vi "FIFORequests.vi"(1 "Log":T1, 3 "Requests in":T1[](array[typedef])) -> (0 "Requests out":T1[](array[typedef]))   [LabVIEW 2010]
uses:
  _ROSDefinition.vi
  Console/Servers/ServerSubs/ROSLog.ctl
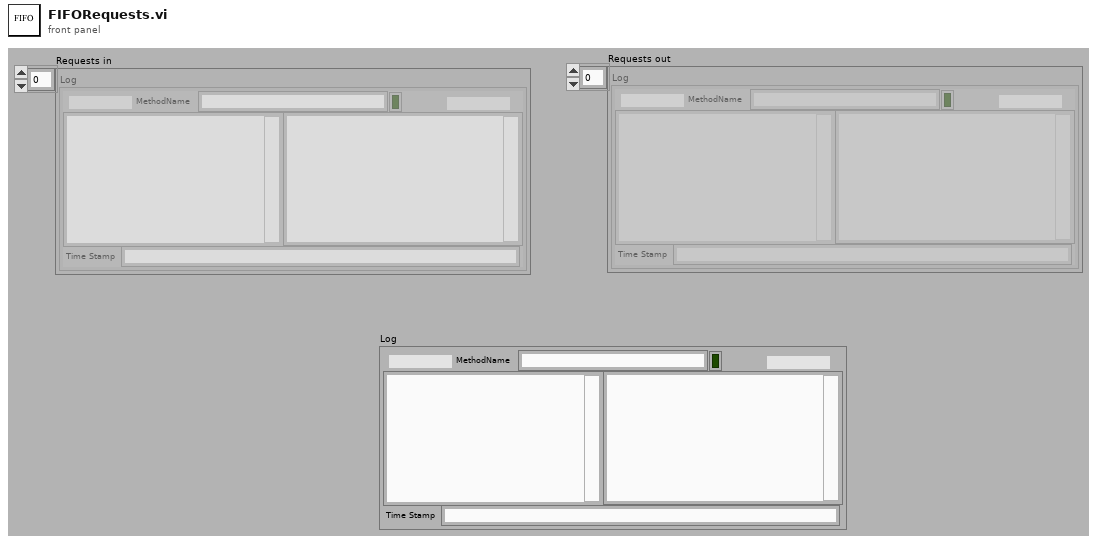
[diagram p1: front panel]
types:
  T1 = typedef "ROSLog.ctl" = cluster{"Sent":string, "Reply":string, "MethodName":string, "success":bool, "Dir1":string, "Dir2":string, "Time Stamp":string}
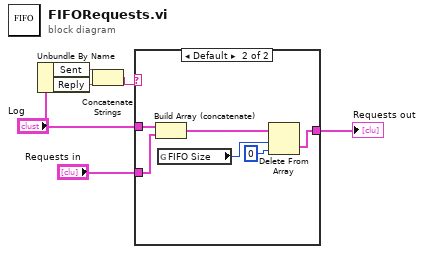
[diagram p0: block diagram]
diagram:
  n1 = Unbundle By Name("Log") -> ("Sent"=w3:string, "Reply"=w2:string)
  n2 = Concatenate Strings(w3, w2) -> (w1:string)
  n3 = case shown="Default" w1 {
    tunnel: "Log" -> [_ w12]
    tunnel: "Requests in" -> [w7 w9]
    tunnel: [w7 w8] -> w5
    frame "" {
    }
    frame Default {
      n4 = Build Array (concatenate)(w12, w9) -> (w13:T1[])
      n5 = global read "_ROSDefinition.vi" "FIFO Size"() -> (w10:i32)
      n6 = Delete From Array(array=w13, length=w10, index=0) -> (deleted portion=w8:T1[])  [unwired: 1 out]
    }
  }
  "Requests out" <- w5
